vi "Build Sequence Array.vi"(6 "Voltage Steps":dbl[](array[numeric])=[8.5, 12.0, 24.0, 36.0, 48.0, 60.0], 9 "Current Sweep Start":dbl=-3.0, 10 "Current Sweep End":dbl, 11 "# Points":i32=50) -> (1 "# Voltage Divisions":i32, 2 "# of Points":i32=50, 3 "To SMU 1 (Source)":dbl[](array[numeric]), 4 "To SMU 2 (Sink)":dbl[](array[numeric]))   [LabVIEW 2014]
uses:
  <vilib>/Analysis/1siggen.llb/Ramp Pattern by Samples.vi
  <vilib>/Analysis/NI_AALBase.lvlib
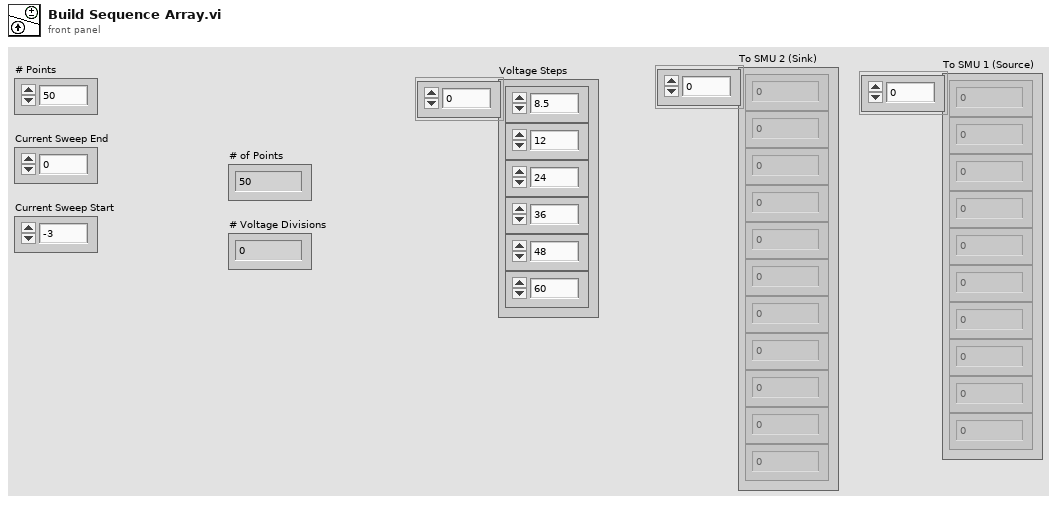
[diagram p1: front panel]
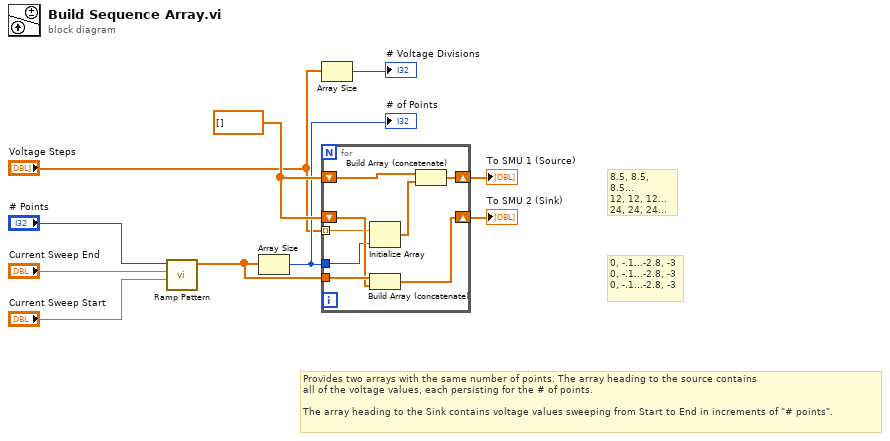
[diagram p0: block diagram]
diagram:
  w10 = dbl[] []
  # "0, -.1...-2.8, -3\n0, -.1...-2.8, -3\n0, -.1...-2.8, -3"
  # "8.5, 8.5, 8.5...\n12, 12, 12...\n24, 24, 24..."
  # "Provides two arrays with the same number of points. The array heading to the source contains \nall of the voltage values, each persisting for the # of points. \n\nThe array heading to the Sink contains voltage values sweeping from Start to End in increments of \"# points\"."
  n1 = call-poly <vilib>:"Ramp Pattern.vi"("start"="Current Sweep Start", "end"="Current Sweep End", "samples"="# Points") -> ("Ramp Pattern"=w5:dbl[])  [unwired: 7 in, 1 out]
  n2 = Array Size(array=w5) -> (size(s)=w7:i32)
  "# of Points" <- w7
  n3 = Array Size(array="Voltage Steps") -> (size(s)=→"# Voltage Divisions":i32)
  n4 = for {
    shift-right: [w16] -> w9
    shift-left: w10 -> [w17]
    shift-right: [w11] -> w8
    shift-left: w10 -> [w12]
    tunnel: w5 -> [w18]
    tunnel: "Voltage Steps" -> [w15] mode=indexing
    tunnel: w7 -> [w14]
    n5 = Initialize Array(w15, w14) -> (w13:dbl[])
    n6 = Build Array (concatenate)(w18, w17) -> (w16:dbl[])
    n7 = Build Array (concatenate)(w12, w13) -> (w11:dbl[])
  }
  "To SMU 2 (Sink)" <- w9
  "To SMU 1 (Source)" <- w8
